vi "CIA1_glb.vi"() -> ()   [LabVIEW 2018]
panel:
  in  "joy2":u8
  in  "IRQ reg":u8
  in  "timer B latch":i32
  in  "timer B":u16
  in  "timer A latch":i32
  out "and matrix":u8 format="%.0x"
  out "key matrix":u8[](array[numeric]) format="%.0x"
  in  "timer A":u16
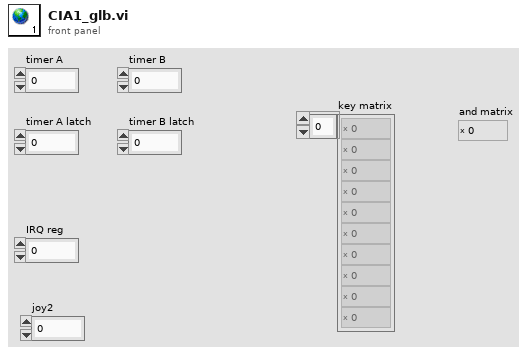
[diagram p1: front panel]
diagram:
